vi "Lockin.Low Pass Filter Bank.vi"(8 "error in (no error)":errorcluster, 10 "WFms in":waveform(dbl)[](array[waveform]), 11 "Instrument.DAQ in":refnum<class "Instrument.DAQ.lvclass">) -> (0 "error out":errorcluster, 2 "Wfms out":waveform(dbl)[](array[waveform]))   [LabVIEW 2019, in "Instrument.DAQ.lvclass"]
uses:
  Instrument.DAQ.lvclass
  <userlib>/_OpenG.lib/array/array.llb/Search 1D Array (I32)__ogtk.vi
panel:
  out "Instrument.DAQ out":refnum<class "Instrument.DAQ.lvclass">
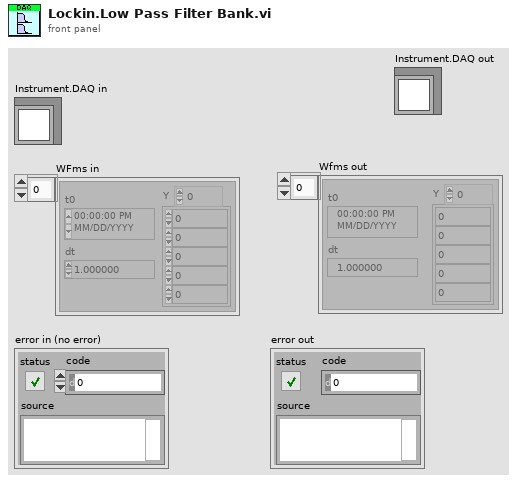
[diagram p1: front panel]
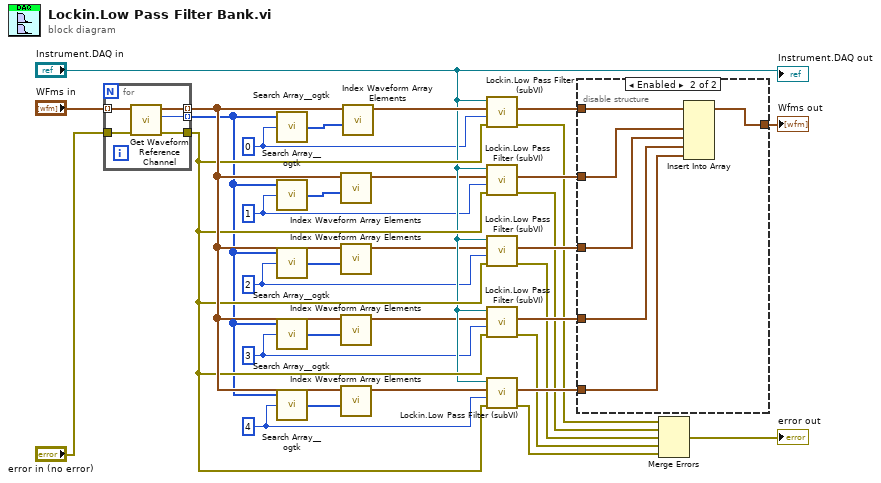
[diagram p0: block diagram]
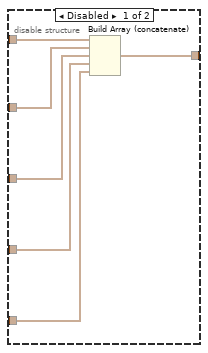
[diagram p2: hidden frame]
diagram:
  w15 = 4 ("Element Data")
  w12 = 3 ("Element Data")
  w13 = 2 ("Element Data")
  w14 = 1 ("Element Data")
  w2 = 0 ("Element Data")
  n1 = for {
    tunnel: [w38] -> w33 mode=indexing
    tunnel: [w37] -> w11 mode=indexing
    tunnel: "WFms in" -> [w36] mode=indexing
    tunnel: "error in (no error)" -> [w35]
    tunnel: [w34] -> w31
    n2 = call "Get Waveform Reference Channel.vi"("error in (no error)"=w35, "Reference in"=w36) -> ("error out"=w34:errorcluster, "Reference Channel"=w37:i32, "Reference out"=w38:waveform(dbl))  [unwired: 7 in]
  }
  n3 = call-poly <userlib>:"Search Array__ogtk.vi"("Array"=w11, "Element Data"=w2) -> ("Indices of Elements"=w30:i32[])  [unwired: 7 in]
  n4 = call-poly <userlib>:"Search Array__ogtk.vi"("Array"=w11, "Element Data"=w14) -> ("Indices of Elements"=w3:i32[])  [unwired: 7 in]
  n5 = call-poly <userlib>:"Search Array__ogtk.vi"("Array"=w11, "Element Data"=w13) -> ("Indices of Elements"=w6:i32[])  [unwired: 7 in]
  n6 = call-poly <userlib>:"Search Array__ogtk.vi"("Array"=w11, "Element Data"=w12) -> ("Indices of Elements"=w7:i32[])  [unwired: 7 in]
  n7 = call-poly <userlib>:"Search Array__ogtk.vi"("Array"=w11, "Element Data"=w15) -> ("Indices of Elements"=w10:i32[])  [unwired: 7 in]
  n8 = call "Index Waveform Array Elements.vi"("Indices of Elements"=w3, "Array in"=w33) -> ("Array out"=w4:waveform(dbl)[])  [unwired: 9 in]
  n9 = call "Index Waveform Array Elements.vi"("Indices of Elements"=w6, "Array in"=w33) -> ("Array out"=w5:waveform(dbl)[])  [unwired: 9 in]
  n10 = call "Index Waveform Array Elements.vi"("Indices of Elements"=w7, "Array in"=w33) -> ("Array out"=w8:waveform(dbl)[])  [unwired: 9 in]
  n11 = call "Index Waveform Array Elements.vi"("Indices of Elements"=w10, "Array in"=w33) -> ("Array out"=w9:waveform(dbl)[])  [unwired: 9 in]
  n12 = call "Index Waveform Array Elements.vi"("Indices of Elements"=w30, "Array in"=w33) -> ("Array out"=w32:waveform(dbl)[])  [unwired: 9 in]
  n13 = call "Lockin.Low Pass Filter (subVI).vi"("error in (no error)"=w31, "Element Data"=w2, "Array"=w32, "Lockin.DAQ in"="Instrument.DAQ in") -> ("error out"=w16:errorcluster, "signal out"=w22:waveform(dbl)[])  [unwired: 5 in, 1 out]
  n14 = call "Lockin.Low Pass Filter (subVI).vi"("error in (no error)"=w31, "Element Data"=w14, "Array"=w4, "Lockin.DAQ in"="Instrument.DAQ in") -> ("error out"=w20:errorcluster, "signal out"=w23:waveform(dbl)[])  [unwired: 5 in, 1 out]
  n15 = call "Lockin.Low Pass Filter (subVI).vi"("error in (no error)"=w31, "Element Data"=w13, "Array"=w5, "Lockin.DAQ in"="Instrument.DAQ in") -> ("error out"=w19:errorcluster, "signal out"=w24:waveform(dbl)[])  [unwired: 5 in, 1 out]
  n16 = call "Lockin.Low Pass Filter (subVI).vi"("error in (no error)"=w31, "Element Data"=w12, "Array"=w8, "Lockin.DAQ in"="Instrument.DAQ in") -> ("error out"=w18:errorcluster, "signal out"=w25:waveform(dbl)[])  [unwired: 5 in, 1 out]
  n17 = call "Lockin.Low Pass Filter (subVI).vi"("error in (no error)"=w31, "Element Data"=w15, "Array"=w9, "Lockin.DAQ in"="Instrument.DAQ in") -> ("error out"=w17:errorcluster, "signal out"=w26:waveform(dbl)[])  [unwired: 5 in, 1 out]
  n18 = disable-structure shown="Enabled" {
    disable-tunnel: [w44 w48] -> w27
    disable-tunnel: w26 -> [w43 w45]
    disable-tunnel: w25 -> [w42 w46]
    disable-tunnel: w24 -> [w41 w47]
    disable-tunnel: w23 -> [w40 w49]
    disable-tunnel: w22 -> [w39 w50]
    frame Disabled {
      n19 = Build Array (concatenate)(w39, w40, w41, w42, w43) -> (w44:waveform(dbl)[])
    }
    frame Enabled {
      n20 = Insert Into Array(array=w50, new element #1=w49, new element #2=w47, new element #3=w46, new element #4=w45) -> (w48:waveform(dbl)[])  [unwired: 1 in]
    }
  }
  "Wfms out" <- w27
  n21 = Merge Errors(w16, w20, w19, w18, w17) -> (→"error out":errorcluster)
  "Instrument.DAQ out" <- "Instrument.DAQ in"
